vi "Get current pretomo stack.vi"(8 "error in (no error)":errorcluster, 11 "Tomo in":refnum<class "Tomo.lvclass">) -> (0 "error out":errorcluster, 1 "y loop number":i32, 2 "x loop number":i32, 3 "Tomo out":refnum<class "Tomo.lvclass">, 4 "z step number":i32)   [LabVIEW 2012, in "Tomo.lvclass"]
uses:
  Tomo.lvclass
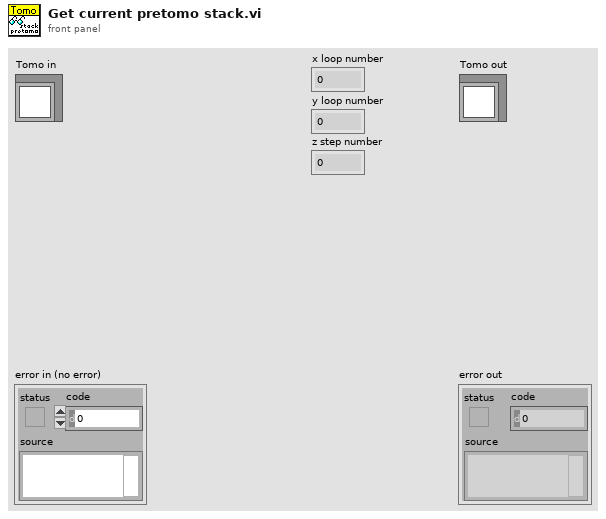
[diagram p1: front panel]
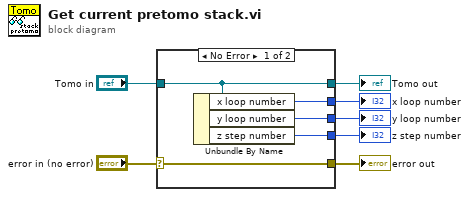
[diagram p0: block diagram]
diagram:
  n1 = case shown="No Error" "error in (no error)" {
    selector: "error in (no error)" -> [w12 w14]
    tunnel: [w12 w14] -> w6
    tunnel: [w11 w13] -> w4
    tunnel: "Tomo in" -> [w11 w13]
    tunnel: [w10 _] -> w3
    tunnel: [w9 _] -> w2
    tunnel: [w8 _] -> w1
    frame No Error {
      n2 = Unbundle By Name(w11) -> ("x loop number"=w10:i32, "y loop number"=w9:i32, "z step number"=w8:i32)
    }
    frame Error {
    }
  }
  "error out" <- w6
  "Tomo out" <- w4
  "x loop number" <- w3
  "y loop number" <- w2
  "z step number" <- w1
